vi "Read Delimited File into VI.vi"() -> ()   [LabVIEW 2020]
uses:
  <vilib>/Utility/file.llb/Read Delimited Spreadsheet (string).vi
  <vilib>/Utility/file.llb/Read Delimited Spreadsheet (DBL).vi
panel:
  out "Waveform Graph":dbl[][](graph)
  out "Data with first line header deleted":dbl[][](array[numeric])
  out "First row (header string)":string[](array[string])
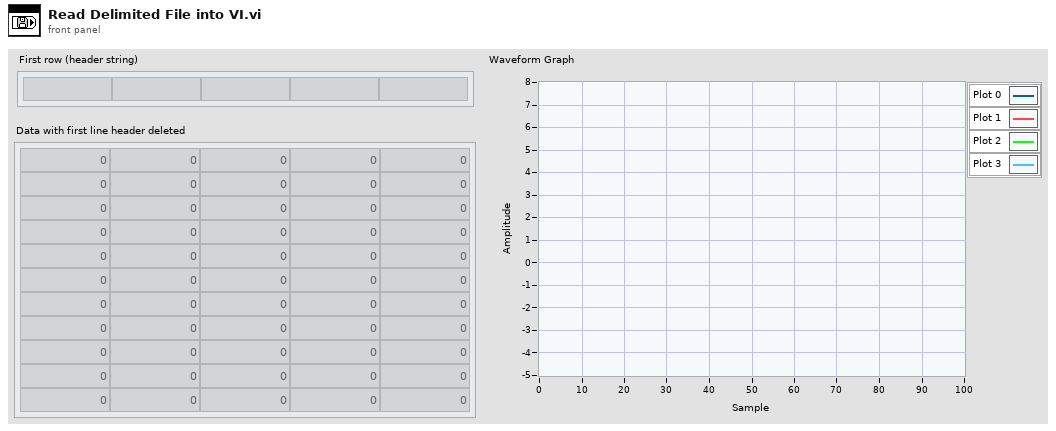
[diagram p1: front panel]
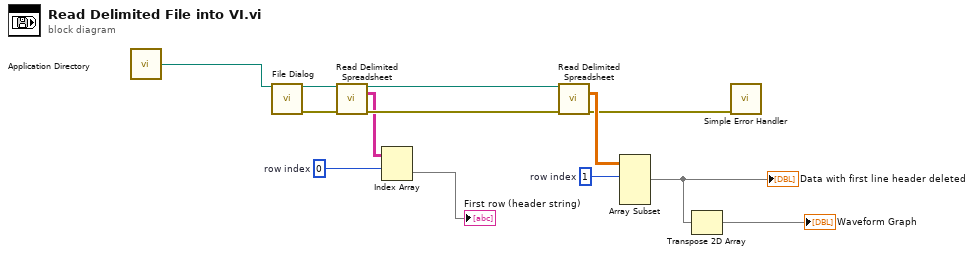
[diagram p0: block diagram]
diagram:
  w5 = 1  # row index
  w7 = 0  # row index
  n1 = call <vilib>:"Application Directory.vi"() -> ("Application Directory"=w13:path)
  n2 = call "File Dialog"("start path"=w13) -> ("selected path"=w12:path, "error out"=w11:errorcluster)  [unwired: 11 in, 2 out]
  n3 = call-poly <vilib>:"Read Delimited Spreadsheet.vi"("file path (dialog if empty)"=w12, "error in (no error)"=w11) -> ("new file path (Not A Path if cancelled)"=w10:path, "all rows"=w8:string[][], "error out"=w9:errorcluster)  [unwired: 8 in, 3 out]
  n4 = Index Array "Index Array"(array=w8, index (row)=w7) -> (element=→"First row (header string)":string[])  [unwired: 1 in]
  n5 = call-poly <vilib>:"Read Delimited Spreadsheet.vi"("file path (dialog if empty)"=w10, "error in (no error)"=w9) -> ("all rows"=w6:dbl[][], "error out"=w1:errorcluster)  [unwired: 8 in, 4 out]
  n6 = Array Subset "Array Subset"(array=w6, index (row)=w5) -> (w2:dbl[][])  [unwired: 3 in]
  "Data with first line header deleted" <- w2
  n7 = Transpose 2D Array(2D array=w2) -> (transposed array=→"Waveform Graph":dbl[][])
  n8 = call <vilib>:"Simple Error Handler.vi"("error in (no error)"=w1) -> ()  [unwired: 4 in, 5 out]
